vi "Own_Code3_AR.vi"() -> ()   [LabVIEW 2012]
uses:
  SubVIs/LVPresent_Globals.vi
panel:
  in  "Tab Control":enum32{"Page 1", "Page 2", "Page 3"}(tab)
  in  "Circuit":bool
  in  "Hint/Solution":bool
  in  "Open":bool
  in  "Back":bool
  in  "Solution":bool
  in  "Back2":bool
  # "Now let's do one more...\n\nFor our last bit of code, let's make a program that turns the LED on and off based on a reading given by the light sensor. Click the button below to start a new VI, and the red button to see the circuit layout. Make sure that you include a loop so that your code runs forever."
  # "Hint: I would use a case structure for this one. Remember to use the help button if you don't know how to use the case structure.\n\n\nThe picture to the right might help too.  Remember that the light sensor\nreads information while the LEDs write information.\n\nYou're also going to need to recognize that the light sensor outputs a \ncertain voltage, which you will use to determine whether the light is on \nor off. To see this voltage, use the Probe Data tool."
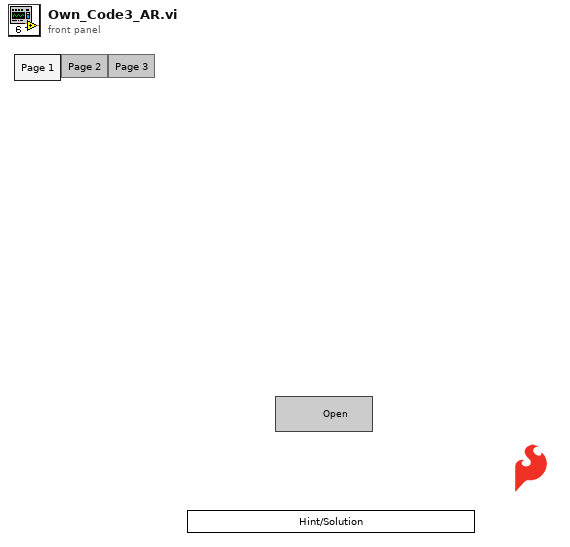
[diagram p1: front panel]
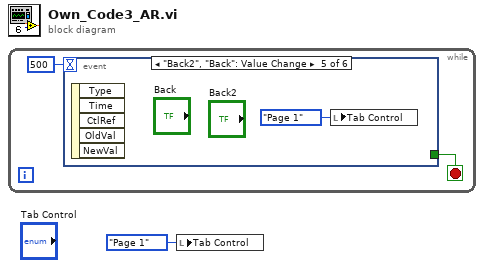
[diagram p0: block diagram]
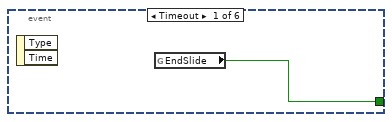
[diagram p2: hidden frame]
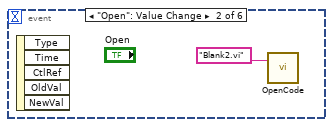
[diagram p3: hidden frame]
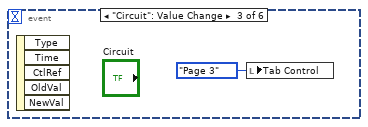
[diagram p4: hidden frame]
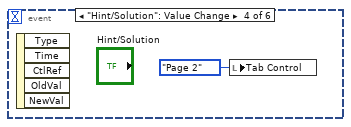
[diagram p5: hidden frame]
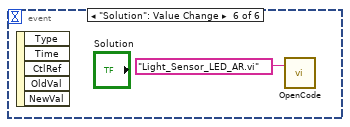
[diagram p6: hidden frame]
diagram:
  n1 = while {
    stop <- w3 stop-if-true
    n2 = event shown="[4] \"Back2\", \"Back\": Value Change" {
      selector: _ -> [_ _ _ _ _ _]
      dyn-events: _ -> [_ _ _ _ _ _]
      timeout: 500 -> [_ _ _ _ _ _]
      tunnel: [w4 _ _ _ _ _] -> w3
      event Timeout {
        n3 = event-data() -> ()  [unwired: 1 in, 2 out]
        n4 = global read "LVPresent_Globals.vi" "EndSlide"() -> (w4:bool)
      }
      event "Open": Value Change {
        n5 = event-data() -> ()  [unwired: 1 in, 5 out]
        n6 = call "OpenCode.vi"("Code name"="Blank2.vi") -> ()  [unwired: 3 in]
      }
      event "Circuit": Value Change {
        n7 = event-data() -> ()  [unwired: 1 in, 5 out]
        n8 = local write "Tab Control"(enum32{"Page 1", "Page 2", "Page 3"}."Page 3" ("Tab Control")) -> ()
      }
      event "Hint/Solution": Value Change {
        n9 = event-data() -> ()  [unwired: 1 in, 5 out]
        n10 = local write "Tab Control"(enum32{"Page 1", "Page 2"}."Page 2" ("Tab Control")) -> ()
      }
      event "Back2", "Back": Value Change {
        n11 = event-data() -> ()  [unwired: 1 in, 5 out]
        n12 = local write "Tab Control"(enum32{"Page 1", "Page 2"}."Page 1" ("Tab Control")) -> ()
      }
      event "Solution": Value Change {
        n13 = event-data() -> ()  [unwired: 1 in, 5 out]
        n14 = call "OpenCode.vi"("Code name"="Light_Sensor_LED_AR.vi") -> ()  [unwired: 3 in]
      }
    }
  }
  n15 = local write "Tab Control"(enum32{"Page 1", "Page 2"}."Page 1" ("Tab Control")) -> ()
